vi "DAC Configure FP View.vi"(8 "error in":errorcluster, 11 "DAC TEG Temp in":refnum<class "DAC TEG Temp.lvclass">) -> (0 "error out":errorcluster, 3 "DAC TEG Temp out":refnum<class "DAC TEG Temp.lvclass">)   [LabVIEW 2019, in "DAC.lvlib" / "DAC TEG Temp.lvclass"]
uses:
  DAC TEG Temp.lvclass
  DAC TEG Temp.lvclass/DAC TEG Temp.ctl
  Results/Heat Flow Results/Heat Flow Results.lvclass/Heat Flow Results.ctl
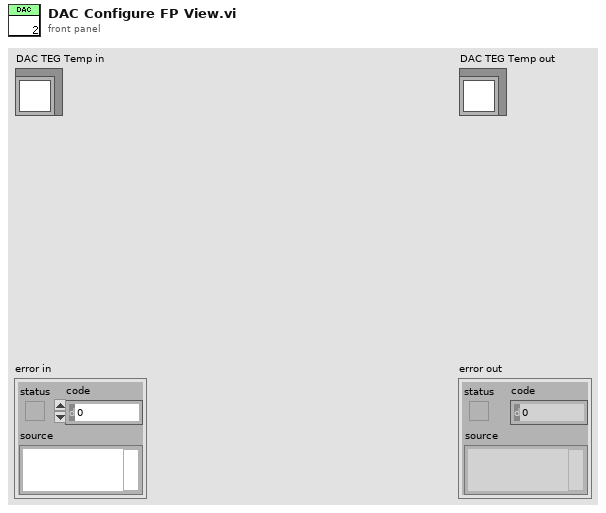
[diagram p1: front panel]
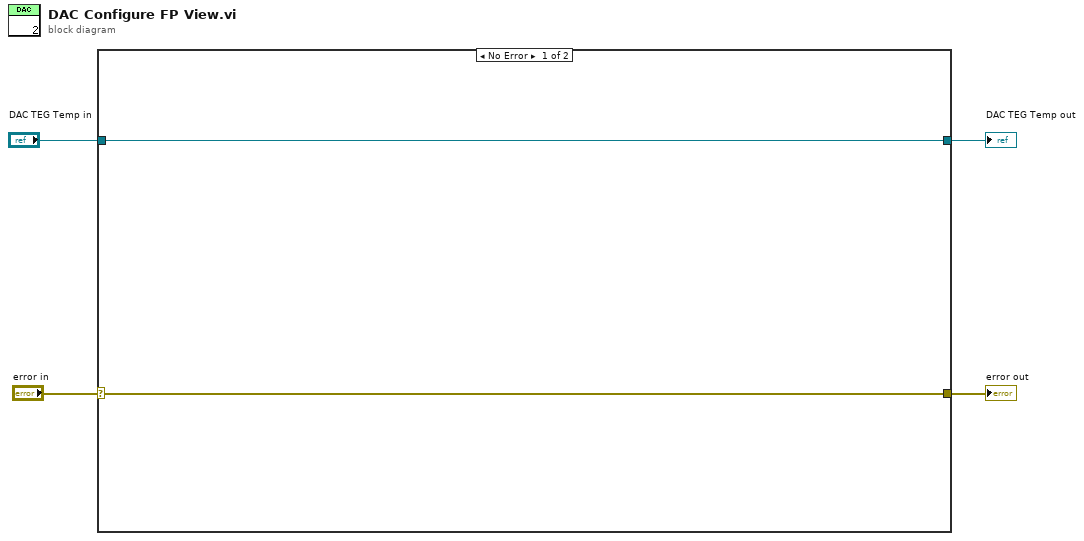
[diagram p0: block diagram]
diagram:
  n1 = case shown="No Error" "error in" {
    selector: "error in" -> [w5 w8]
    tunnel: [w5 w8] -> w1
    tunnel: [w6 w7] -> w2
    tunnel: "DAC TEG Temp in" -> [w6 w7]
    frame No Error {
    }
    frame Error {
    }
  }
  "error out" <- w1
  "DAC TEG Temp out" <- w2
